vi "UE9 Stream with Stream-DAC and SPI.vi"() -> ()   [LabVIEW 2021]
panel:
  out "SPI error":errorcluster
  out "stream error":errorcluster
  in  "U8 Array Write":u8[](array[numeric])=[170, 240, 170, 240]
  out "U8 Array Read":u8[](array[numeric])
  in  "# Bytes To Transfer (1-50)":i32=4 min=1 max=50
  in  "DAC1 # Update Points (0-128":i32=2
  in  "DAC0 # Update Points (0-128)":i32=10
  in  "DAC Data":dbl[][](array[numeric])=[[0.0, 0.0], [1.0, 5.0], [2.0, 0.0], [3.0, 0.0], [4.0, 0.0], [5.0, 0.0], [4.0, 0.0], [3.0, 0.0], [2.0, 0.0], [1.0, 0.0]] format="%.3f"
  out "Actual Scan Rate (Hz)":dbl=1000.0 format="%.3f"
  out "# Scans Read":i32
  out "# of iterations":i32
  out "AIN0 Data":dbl[](array[numeric]) format="%.3f"
  in  "Scan Rate (Hz)":dbl=1000.0 format="%.3f"
  in  "stop":bool
  out "Error Message":string
  # "This example streams from AIN0 using the\nfirst found USB UE9.  Updates both DACs\nat the same rate.\n\nRequires Control firmware V1.94 or higher."
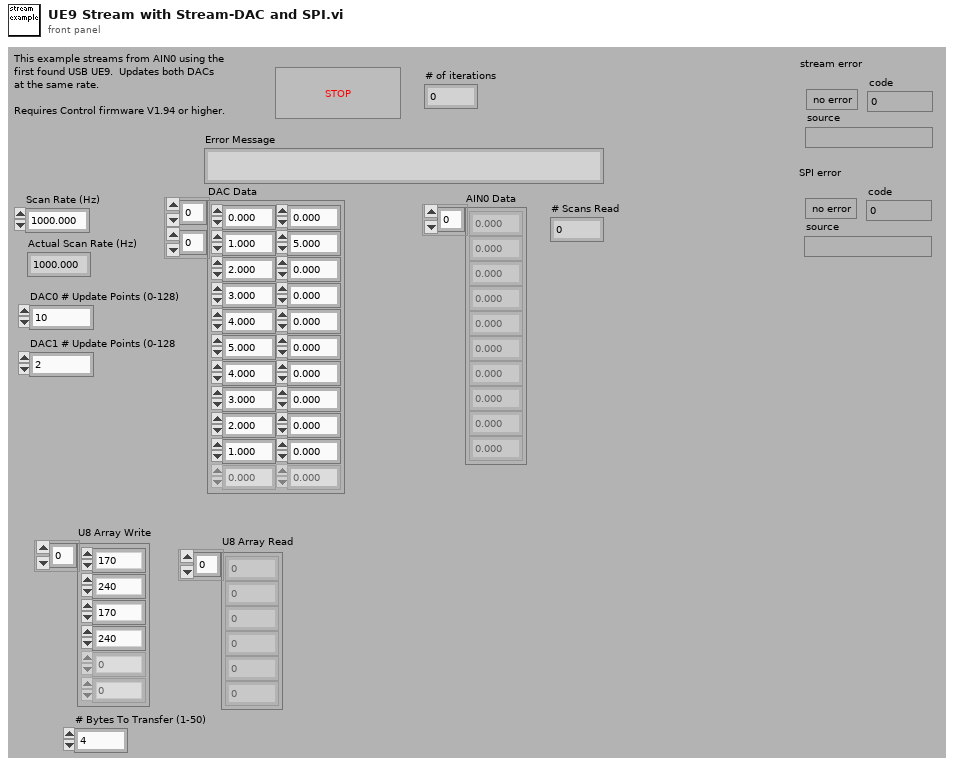
[diagram p1: front panel]
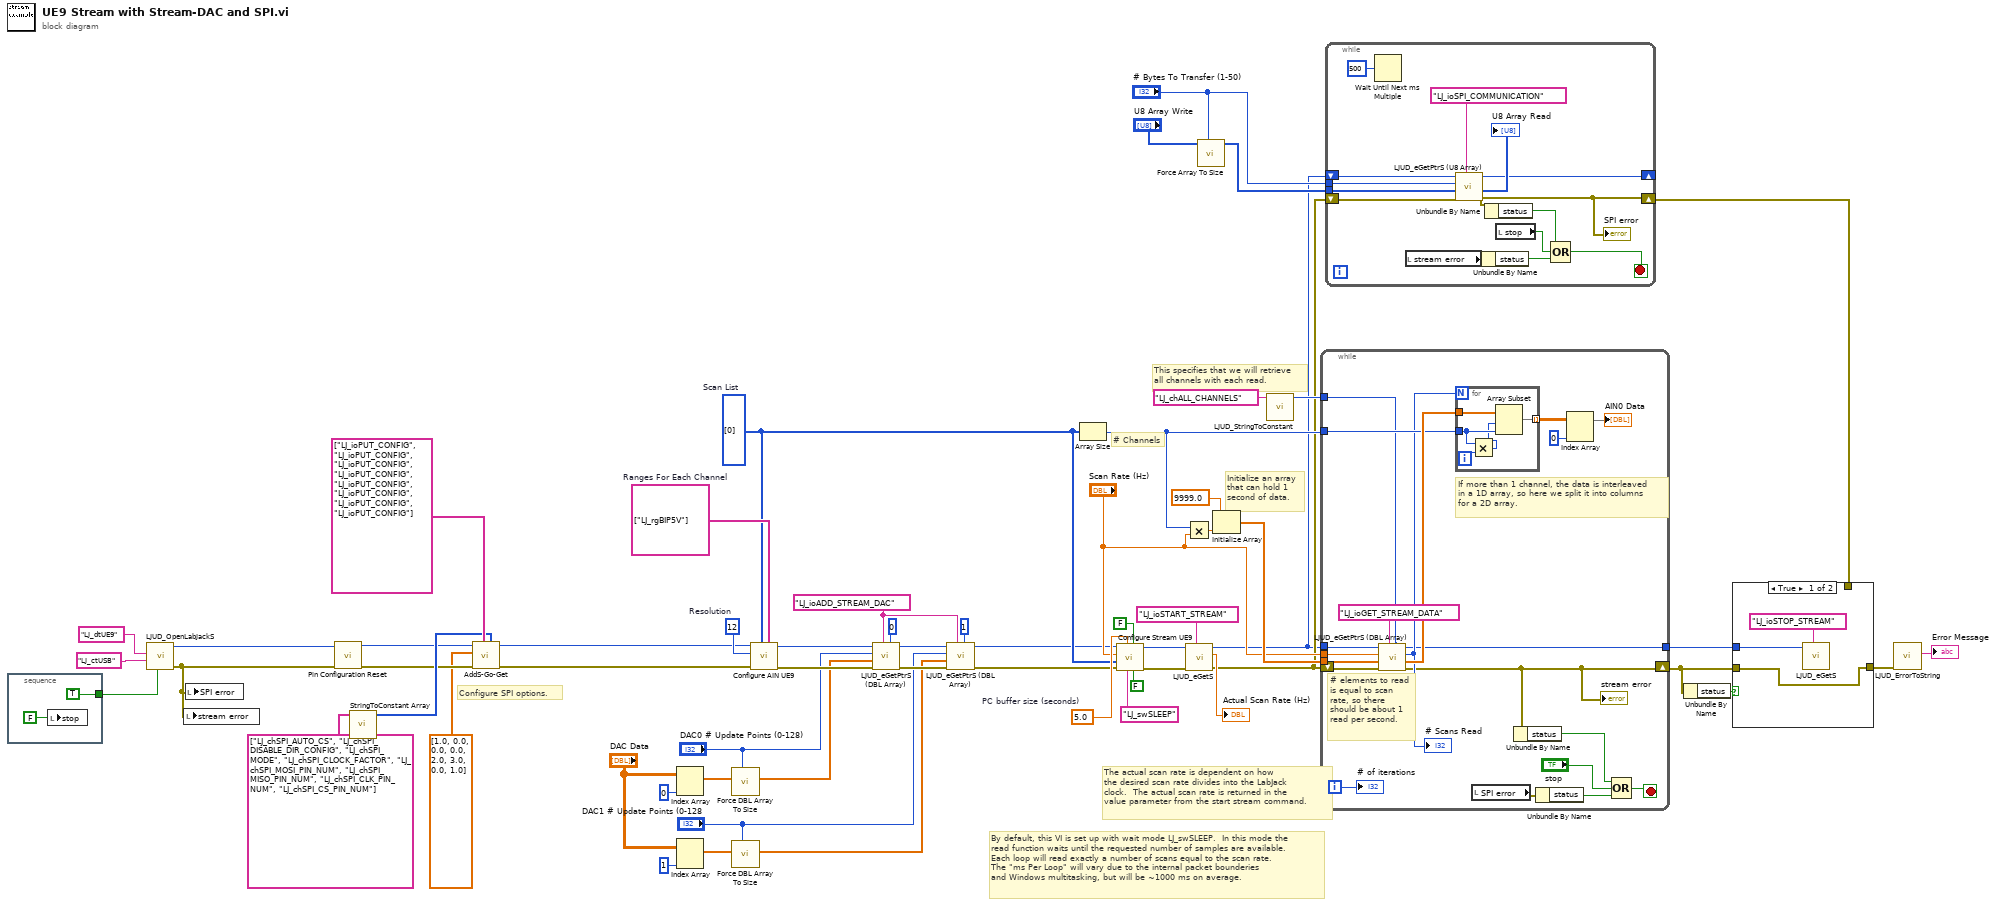
[diagram p0: block diagram]
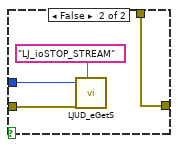
[diagram p2: hidden frame]
diagram:
  w18 = "LJ_ioADD_STREAM_DAC" ("IOType")
  w39 = 12  # Resolution
  w40 = i32[] [0]  # Scan List
  w41 = string[] ["LJ_rgBIP5V"]  # Ranges For Each Channel
  w49 = 5.0  # PC buffer size (seconds)
  # "Configure SPI options."
  # "Initialize an array\nthat can hold 1\nsecond of data."
  # "# Channels"
  # "This specifies that we will retrieve\nall channels with each read."
  # "The actual scan rate is dependent on how\nthe desired scan rate divides into the LabJack\nclock.  The actual scan rate is returned in the\nvalue parameter from the start stream command."
  # "By default, this VI is set up with wait mode LJ_swSLEEP.  In this mode the\nread function waits until the requested number of samples are available.\nEach loop will read exactly a number of scans equal to the scan rate.\nThe \"ms Per Loop\" will vary due to the internal packet bounderies\nand Windows multitasking, but will be ~1000 ms on average."
  n1 = stacked-sequence {
    tunnel: [TRUE ("FirstFound")] -> w1
    frame #0 {
      n2 = local write "stop"(FALSE ("stop")) -> ()
    }
  }
  n3 = call "LJUD_OpenLabJackS.vi"("FirstFound"=w1, "ConnectionType"="LJ_ctUSB", "DeviceType"="LJ_dtUE9") -> ("error out"=w2:errorcluster, "Handle"=w3:i32)  [unwired: 6 in, 1 out]
  n4 = local write "stream error"(w2) -> ()
  n5 = local write "SPI error"(w2) -> ()
  n6 = call "Pin Configuration Reset.vi"("error in"=w2, "Handle In"=w3) -> ("error out"=w14:errorcluster, "Handle Out"=w15:i32)  [unwired: 8 in]
  n7 = call "StringToConstant Array.vi"("String Constant Array In"=string[] ["LJ_chSPI_AUTO_CS", "LJ_chSPI_DISABLE_DIR_CONFIG", "LJ_chSPI_MODE", "LJ_chSPI_CLOCK_FACTOR", "LJ_chSPI_MOSI_PIN_NUM", "LJ_chSPI_MISO_PIN_NUM", "LJ_chSPI_CLK_PIN_NUM", "LJ_chSPI_CS_PIN_NUM"] ("IOTypes")) -> ("I32 Constant Array Out"=w16:i32[])  [unwired: 10 in]
  n8 = call "AddS-Go-Get.vi"("Channels"=w16, "IOTypes"=string[] ["LJ_ioPUT_CONFIG", "LJ_ioPUT_CONFIG", "LJ_ioPUT_CONFIG", "LJ_ioPUT_CONFIG", "LJ_ioPUT_CONFIG", "LJ_ioPUT_CONFIG", "LJ_ioPUT_CONFIG", "LJ_ioPUT_CONFIG"], "error in"=w14, "Values Write"=dbl[] [1.0, 0.0, 0.0, 0.0, 2.0, 3.0, 0.0, 1.0], "Handle In"=w15) -> ("error out"=w8:errorcluster, "Handle Out"=w7:i32)  [unwired: 4 in, 1 out]
  n9 = Index Array(array="DAC Data", index (col)=0 ("Disabled Index (col)")) -> (element=w35:dbl[])  [unwired: 1 in]
  n10 = Index Array(array="DAC Data", index (col)=1 ("Disabled Index (col)")) -> (element=w34:dbl[])  [unwired: 1 in]
  n11 = call "Force DBL Array To Size.vi"("# Elements"="DAC0 # Update Points (0-128)", "DBL Array In"=w35) -> ("DBL Array Out"=w26:dbl[])  [unwired: 9 in]
  n12 = call "Force DBL Array To Size.vi"("# Elements"="DAC1 # Update Points (0-128", "DBL Array In"=w34) -> ("DBL Array Out"=w25:dbl[])  [unwired: 9 in]
  n13 = call "Configure AIN UE9.vi"("Ranges"=w41, "Channels"=w40, "error in"=w8, "Resolution"=w39, "Handle In"=w7) -> ("error out"=w30:errorcluster, "Handle Out"=w29:i32)  [unwired: 5 in]
  n14 = call "LJUD_eGetPtrS (DBL Array).vi"("Channel"=0, "IOType"=w18, "error in"=w30, "DBL Array Write"=w26, "Value"="DAC0 # Update Points (0-128)", "Handle In"=w29) -> ("error out"=w27:errorcluster, "Handle Out"=w28:i32)  [unwired: 2 in, 2 out]
  n15 = call "LJUD_eGetPtrS (DBL Array).vi"("Channel"=1, "IOType"=w18, "error in"=w27, "DBL Array Write"=w25, "Value"="DAC1 # Update Points (0-128", "Handle In"=w28) -> ("error out"=w19:errorcluster, "Handle Out"=w20:i32)  [unwired: 2 in, 2 out]
  n16 = Array Size(array=w40) -> (size(s)=w54:i32)
  n17 = call "Configure Stream UE9.vi"("External Scan Trigger"=FALSE, "Scan Clock Output"=FALSE, "Wait Mode"="LJ_swSLEEP" ("Wait Mode (2)"), "PC buffer size (seconds)"=w49, "error in"=w19, "Scan List"=w40, "Scan Rate (Hz)"="Scan Rate (Hz)", "Handle In"=w20) -> ("error out"=w58:errorcluster, "Handle Out"=w59:i32)  [unwired: 1 in, 1 out]
  n18 = Multiply(x=w54, y="Scan Rate (Hz)") -> (x*y=w57:dbl)
  n19 = call "LJUD_eGetS.vi"("IOType"="LJ_ioSTART_STREAM", "error in"=w58, "Handle In"=w59) -> ("error out"=w6:errorcluster, "Value Read"=→"Actual Scan Rate (Hz)":dbl, "Handle Out"=w5:i32)  [unwired: 6 in]
  n20 = call "Force Array To Size.vi"("# Elements"="# Bytes To Transfer (1-50)", "I32 Array In"="U8 Array Write") -> ("I32 Array Out"=w11:i32[])  [unwired: 6 in, 3 out]
  n21 = Initialize Array(9999.0, w57) -> (w55:dbl[])
  n22 = call "LJUD_StringToConstant.vi"("String"="LJ_chALL_CHANNELS") -> ("Constant Number"=w42:i32)  [unwired: 9 in, 1 out]
  n23 = while {
    shift-left: w6 -> [w73]
    shift-right: [w68] -> w36
    tunnel: w42 -> [w75]
    tunnel: [w72] -> w52
    tunnel: w54 -> [w77]
    tunnel: w55 -> [w80]
    tunnel: "Scan Rate (Hz)" -> [w78]
    tunnel: w5 -> [w82]
    i -> [w76]
    stop <- w63 stop-if-true
    # "If more than 1 channel, the data is interleaved\nin a 1D array, so here we split it into columns\nfor a 2D array."
    # "# elements to read\nis equal to scan\nrate, so there\nshould be about 1\nread per second."
    n24 = call "LJUD_eGetPtrS (DBL Array).vi"("Channel"=w75, "IOType"="LJ_ioGET_STREAM_DATA", "error in"=w73, "DBL Array Write"=w80, "Value"=w78, "Handle In"=w82) -> ("error out"=w68:errorcluster, "DBL Array Read"=w79:dbl[], "Value"=w74:i32, "Handle Out"=w72:i32)  [unwired: 2 in]
    "# Scans Read" <- w74
    "stream error" <- w68
    n25 = for {
      N: w74 -> [_]
      tunnel: w79 -> [w87]
      tunnel: w77 -> [w86]
      tunnel: [w83] -> w71 mode=indexing
      i -> [w85]
      n26 = Multiply(x=w86, y=w85) -> (x*y=w84:i32)
      n27 = Array Subset(array=w87, index=w84, length=w86) -> (w83:dbl[])
    }
    n28 = local read "SPI error"() -> (w64:errorcluster)
    n29 = Unbundle By Name(w68) -> ("status"=w66:bool)
    n30 = Unbundle By Name(w64) -> ("status"=w65:bool)
    n31 = Index Array(array=w71, index (col)=0 ("Disabled Index (col)")) -> (element=→"AIN0 Data":dbl[])  [unwired: 1 in]
    n32 = Compound Arithmetic op=OR(w66, "stop", w65) -> (w63:bool)
    "# of iterations" <- w76
  }
  n33 = while {
    shift-left: w5 -> [w95]
    shift-right: [w94] -> _
    shift-left: w6 -> [w96]
    shift-right: [w89] -> w4
    tunnel: "# Bytes To Transfer (1-50)" -> [w100]
    tunnel: w11 -> [w101]
    stop <- w91 stop-if-true
    n34 = Wait Until Next ms Multiple(millisecond multiple=u32 500) -> ()  [unwired: 1 out]
    n35 = local read "stream error"() -> (w88:errorcluster)
    n36 = call "LJUD_eGetPtrS (U8 Array).vi"("IOType"="LJ_ioSPI_COMMUNICATION", "error in"=w96, "U8 Array Write"=w101, "Value"=w100, "Handle In"=w95) -> ("error out"=w89:errorcluster, "U8 Array Read"=→"U8 Array Read":u8[], "Handle Out"=w94:i32)  [unwired: 3 in, 1 out]
    "SPI error" <- w89
    n37 = Unbundle By Name(w88) -> ("status"=w90:bool)
    n38 = Unbundle By Name(w89) -> ("status"=w93:bool)
    n39 = local read "stop"() -> (w92:bool)
    n40 = Compound Arithmetic op=OR(w93, w92, w90) -> (w91:bool)
  }
  n41 = Unbundle By Name(w36) -> ("status"=w44:bool)
  n42 = case shown="True" w44 {
    tunnel: w52 -> [w103 w107]
    tunnel: [w102 w105] -> w51
    tunnel: w36 -> [w102 w106]
    tunnel: w4 -> [_ w105]
    frame True {
      n43 = call "LJUD_eGetS.vi"("IOType"="LJ_ioSTOP_STREAM", "Handle In"=w103) -> ()  [unwired: 7 in, 3 out]
    }
    frame False {
      n44 = call "LJUD_eGetS.vi"("IOType"="LJ_ioSTOP_STREAM", "error in"=w106, "Handle In"=w107) -> ()  [unwired: 6 in, 3 out]
    }
  }
  n45 = call "LJUD_ErrorToString.vi"("error in"=w51) -> ("String"=→"Error Message":string)  [unwired: 10 in]
